vi "IL-RL Standards.vi"(10 "Input New Standard":T1) -> (2 "IL RL Standards":T2(array[cluster])=[{"Standard Name"="GR326-UPC-New ", "Max IL to Pass (dB)"=0.4, "Min RL to Pass (dB)"=40.0}, {"Standard Name"="GR326-UPC-During/End", "Max IL to Pass (dB)"=0.5, "Min RL to Pass (dB)"=40.0}, {"Standard Name"="GR326-APC-New ", "Max IL to Pass (dB)"=0.4, "Min RL to Pass (dB)"=60.0}, {"Standard Name"="GR326-APC-During/End", "Max IL to Pass (dB)"=0.5, "Min RL to Pass (dB)"=60.0}, {"Standard Name"="GR1435-Standard-New", "Max IL to Pass (dB)"=0.7, "Min RL to Pass (dB)"=-55.0}, {"Standard Name"="GR1435-Standard-During/End", "Max IL to Pass (dB)"=0.8, "Min RL to Pass (dB)"=-50.0}], 3 "Standard Names":string[](array[string])=["Select Test Standard", "---------------------", "No Standard", "Custom Standard", "---------------------", "GR326-UPC-New ", "GR326-UPC-During/End", "GR326-APC-New ", "GR326-APC-During/End", "GR1435-Standard-New", "GR1435-Standard-During/End"])   [LabVIEW 2017]
panel:
  out "Standard Ring":u16(ring) items=["GR326-UPC-New ", "GR326-UPC-During/End", "GR326-APC-New ", "GR326-APC-During/End", "GR1435-Standard-New", "GR1435-Standard-During/End"]
  # "Add new Standard\n1) Add new Standard into \"Input New Standard\"\n2) Run program\n3) Edit > \"Make current values default\""
  # "Delete old Standard\n1) Right click cluster in array with old standard\n2) Data Operations > \"Delete Element\"\n3) Run program\n4) Edit > \"Make current values default\""
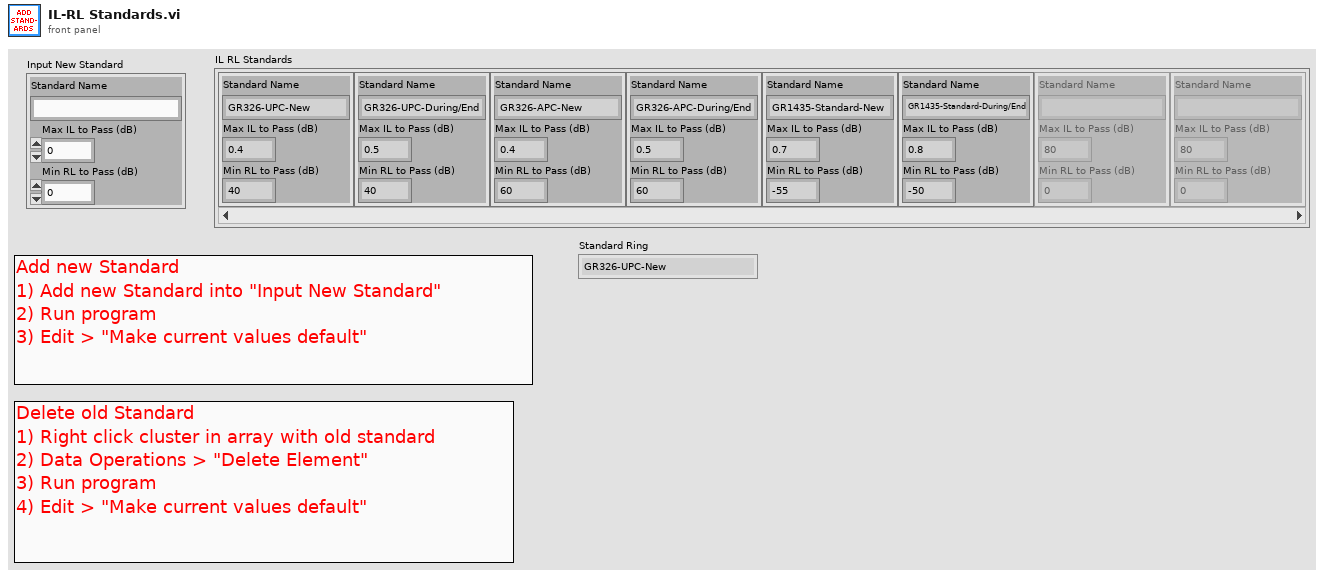
[diagram p1: front panel]
types:
  T1 = cluster{"Standard Name":string, "Max IL to Pass (dB)":dbl, "Min RL to Pass (dB)":dbl}
  T2 = cluster{"Standard Name":string, "Max IL to Pass (dB)":dbl, "Min RL to Pass (dB)":dbl}[]
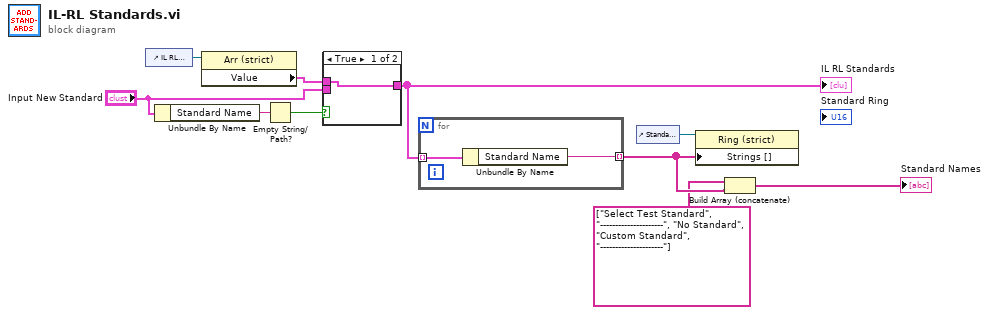
[diagram p0: block diagram]
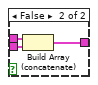
[diagram p2: hidden frame]
diagram:
  n1 = control-ref of="IL RL Standards"() -> (w10:refnum<vi>)
  n2 = Unbundle By Name("Input New Standard") -> ("Standard Name"=w5:string)
  n3 = property class="Arr (strict)"(reference=w10) -> ("Value"=w9:T2)  [unwired: 1 in, 2 out]
  n4 = Empty String/Path?(string/path=w5) -> (empty?=w4:bool)
  n5 = case shown="True" w4 {
    tunnel: w9 -> [w11 w14]
    tunnel: "Input New Standard" -> [_ w13]
    tunnel: [w11 w12] -> w8
    frame True {
    }
    frame False {
      n6 = Build Array (concatenate)(w14, w13) -> (w12:T2)
    }
  }
  "IL RL Standards" <- w8
  n7 = for {
    tunnel: w8 -> [w16] mode=indexing
    tunnel: [w15] -> w3 mode=indexing
    n8 = Unbundle By Name(w16) -> ("Standard Name"=w15:string)
  }
  n9 = control-ref of="Standard Ring"() -> (w7:refnum<vi>)
  n10 = property class="Ring (strict)"(reference=w7, "Strings []"=w3) -> ()  [unwired: 1 in, 2 out]
  n11 = Build Array (concatenate)(string[] ["Select Test Standard", "---------------------", "No Standard", "Custom Standard", "---------------------"] ("new element/subarray"), w3) -> (→"Standard Names":string[])
